vi "Set Shutter.vi"(7 "openingtime":i32, 8 "error in (no error)":errorcluster, 9 "closingtime":i32, 10 "mode":i32, 11 "typ":i32) -> (0 "error out":errorcluster, 3 "function return":u32)   [LabVIEW 2018, in "AndorSDK.lvlib"]
doc: "EXPNETTYPE unsigned int WINAPI SetShutter(int typ, int mode, int closingtime, int openingtime);"
uses:
  AndorSDK.lvlib
  ATMCD32D.dll
  OwnVIs/AndorOWN.lvlib
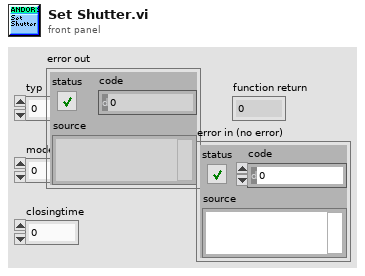
[diagram p1: front panel]
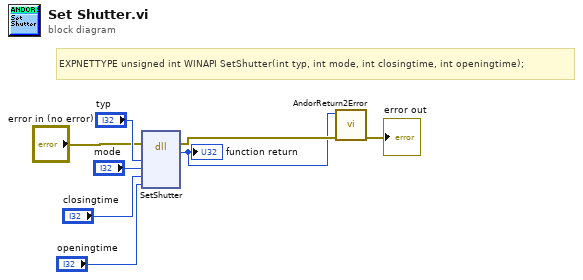
[diagram p0: block diagram]
diagram:
  # "EXPNETTYPE unsigned int WINAPI SetShutter(int typ, int mode, int closingtime, int openingtime);"
  n1 = dll-call lib="C:/Users/e14user/Documents/LabVIEW software/GitRepo/lib/ANDOR/Andor SDK/ATMCD32D.*" fn="SetShutter"(error in="error in (no error)", "typ"="typ", "mode"="mode", "closingtime"="closingtime", "openingtime"="openingtime") -> (error out=w3:errorcluster, w2:u32)  [unwired: 6 in, 1 out]
  "function return" <- w2
  n2 = call "AndorReturn2Error.vi"("error in (no error)"=w3, "Camera return"=w2) -> ("error out"=→"error out":errorcluster)  [unwired: 9 in]
